vi "writeToXML.vi"(8 "error in (no error)":errorcluster, 10 "ClassLabel":string, 11 "GuiderName in":refnum<class "GuiderName.lvclass">) -> (0 "error out":errorcluster, 2 "XMLout":string, 3 "GuiderName out":refnum<class "GuiderName.lvclass">)   [LabVIEW 2014, in "TCSDataDefinitions.lvlib" / "TCSGuiderCommand.lvlib" / "GuiderName.lvclass"]
uses:
  GuiderName.lvclass
  GuiderName.lvclass/GuiderName.ctl
  TCSGuiderCommand/TCSGuiderCommand.lvclass
  <userlib>/Common/XML/XMLGenerator/XMLGenerator.lvclass
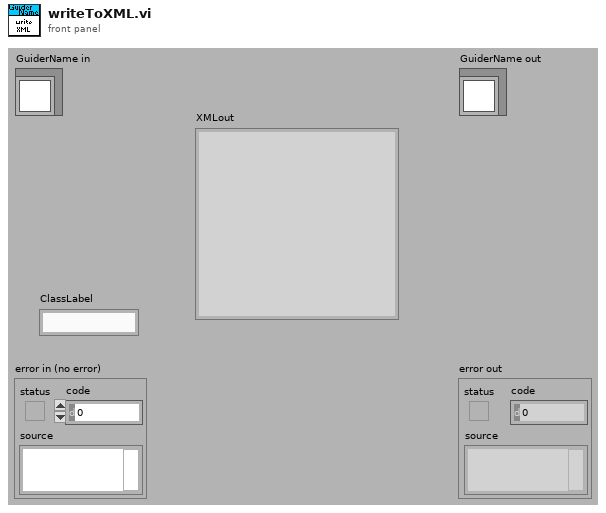
[diagram p1: front panel]
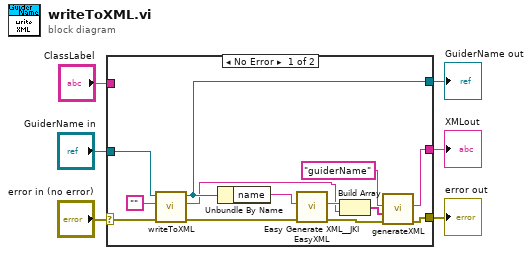
[diagram p0: block diagram]
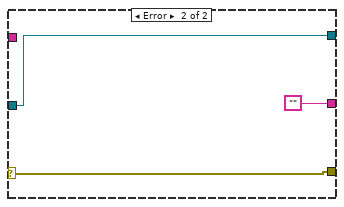
[diagram p2: hidden frame]
diagram:
  n1 = case shown="No Error" "error in (no error)" {
    selector: "error in (no error)" -> [w11 w22]
    tunnel: [w10 w22] -> w5
    tunnel: [w18 w21] -> w3
    tunnel: "GuiderName in" -> [w19 w21]
    tunnel: "ClassLabel" -> [_ _]
    tunnel: [w9 ""] -> w1
    frame No Error {
      n2 = call-parent "writeToXML.vi"("error in (no error)"=w11, "ClassLAbel"="", "TCSGuiderCommand.lvclass"=w19) -> ("error out"=w15:errorcluster, "XML out"=w7:string, "TCSGuiderCommand.lvclass 2"=w18:refnum<class "GuiderName.lvclass">)  [unwired: 6 in]
      n3 = Unbundle By Name(w18) -> ("name"=w16:string)
      n4 = call <vilib>:"Easy Generate XML__JKI EasyXML.vi"("error in (no error)"=w15, "LabVIEW Data"=w16) -> ("error out"=w12:errorcluster, "XML String"=w8:string)  [unwired: 8 in]
      n5 = Build Array(w8, w7) -> (w14:string[])
      n6 = call <userlib>:"generateXML.vi"("error in"=w12, "childrenXML"=w14, "elementName"="guiderName" ("Class Label")) -> ("error out"=w10:errorcluster, "XML out"=w9:string)  [unwired: 6 in, 1 out]
    }
    frame Error {
    }
  }
  "error out" <- w5
  "GuiderName out" <- w3
  "XMLout" <- w1
